vi "UDP Sender.vi"(0 "Ports to Check":T4, 1 "Connection Established?":bool, 3 "error in (no error)":errorcluster) -> (7 "Results":T1, 8 "Test Finished?":bool, 9 "Message from Server":string, 10 "error out":errorcluster)   [LabVIEW 2019]
uses:
  Documents/GitHub/InsightCM-PortChecker/PortChecker/src/controls/Ports to Check.ctl
  Documents/GitHub/InsightCM-PortChecker/PortChecker/src/controls/Results.ctl
  Documents/GitHub/InsightCM-PortChecker/PortChecker/src/controls/Log Data Cluster.ctl
  Documents/GitHub/InsightCM-PortChecker/PortChecker/src/controls/Communication Types.ctl
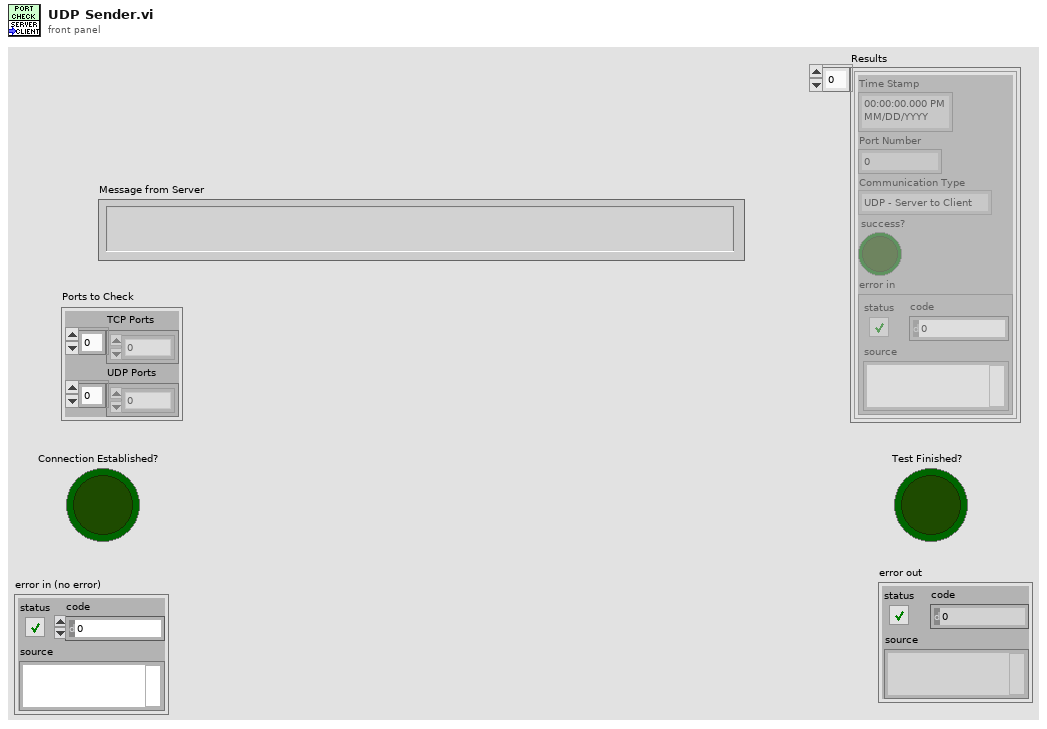
[diagram p1: front panel]
types:
  T1 = typedef "Results.ctl" = T2[]
  T2 = typedef "log data cluster.ctl" = cluster{"Time Stamp":timestamp, "Port Number":u16, "Communication Type":T3, "success?":bool, "error in":errorcluster}
  T3 = typedef "Communication Types.ctl" = enum16{"UDP - Server to Client", "UDP - Client to Server", "TCP - Server to Client", "TCP - Client to Server"}
  T4 = typedef "Ports to Check.ctl" = cluster{"TCP Ports":u16[], "UDP Ports":u16[]}
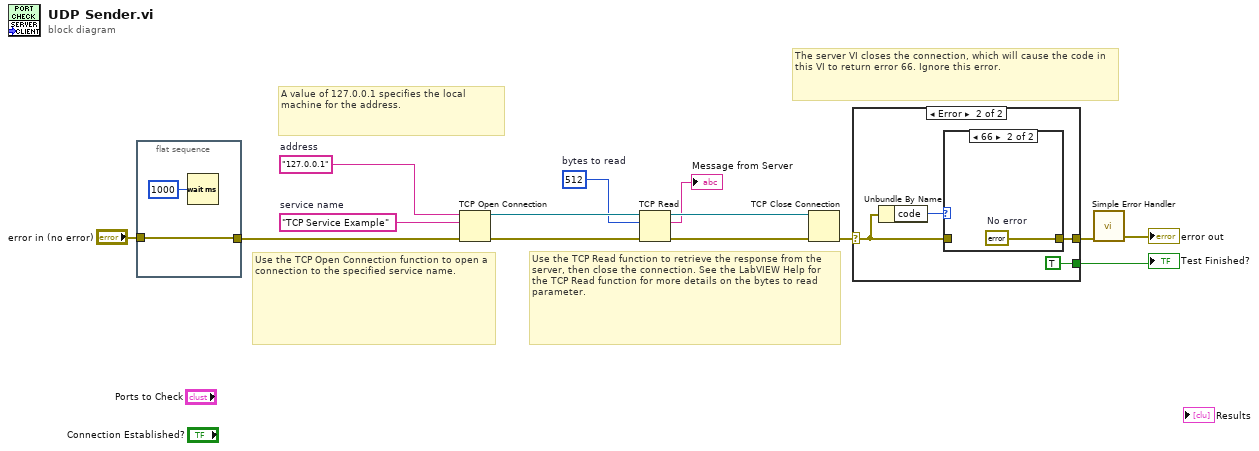
[diagram p0: block diagram]
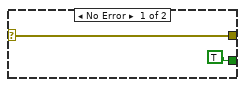
[diagram p2: hidden frame]
diagram:
  w7 = 512  # bytes to read
  w8 = "TCP Service Example"  # service name
  w9 = "127.0.0.1"  # address
  # "The server VI closes the connection, which will cause the code in this VI to return error 66. Ignore this error."
  # "A value of 127.0.0.1 specifies the local machine for the address."
  # "Use the TCP Open Connection function to open a connection to the specified service name."
  # "Use the TCP Read function to retrieve the response from the server, then close the connection. See the LabVIEW Help for the TCP Read function for more details on the bytes to read parameter."
  n1 = flat-sequence {
    tunnel: "error in (no error)" -> [w15]
    tunnel: [w15] -> w1
    frame #0 {
      n2 = Wait (ms)(milliseconds to wait=u32 1000) -> ()  [unwired: 1 out]
    }
  }
  n3 = TCP Open Connection(address=w9, remote port or service name=w8, error in (no error)=w1) -> (connection ID=w13:refnum<k5>, error out=w14:errorcluster)  [unwired: 2 in]
  n4 = TCP Read(connection ID=w13, bytes to read=w7, error in (no error)=w14) -> (connection ID out=w12:refnum<k5>, data out=→"Message from Server":string, error out=w11:errorcluster)  [unwired: 2 in]
  n5 = TCP Close Connection(connection ID=w12, error in (no error)=w11) -> (error out=w6:errorcluster)  [unwired: 1 in, 1 out]
  n6 = case shown="Error" w6 {
    selector: w6 -> [w18 w21]
    tunnel: [w18 w20] -> w5
    tunnel: [TRUE TRUE] -> w3
    frame No Error {
    }
    frame Error {
      n7 = Unbundle By Name(w21) -> ("code"=w22:i32)
      n8 = case shown="66" w22 {
        tunnel: w21 -> [w23 _]
        tunnel: [w23 w24] -> w20
        frame Default {
        }
        frame 66 {
          w24 = errorcluster {"status"=FALSE, "code"=0, "source"=""}  # No error
        }
      }
    }
  }
  "Test Finished?" <- w3
  n9 = call <vilib>:"Simple Error Handler.vi"("error in (no error)"=w5) -> ("error out"=→"error out":errorcluster)  [unwired: 4 in, 4 out]
